vi "Panel DPT Channel Test Labels.vi"(5 "CDAQ?":bool) -> (6 "Chanel List":string="1001,1002,1003", 8 "Label Array":string[](array[string])=["RDB F", "Room Ambient(F)", "Tscale"], 10 "Pannel Array":string[](array[string])=["1-1", "1-2", "1-3"])   [LabVIEW 2012]
uses:
  DPT Channel Label.ctl
  <vilib>/Utility/file.llb/Write To Spreadsheet File (string).vi
  <vilib>/Utility/file.llb/Read From Spreadsheet File (string).vi
panel:
  out "error out":errorcluster={"status"=TRUE, "code"=1, "source"="Set Permissions in Panel DPT Channel Test Labels.vi<APPEND>\n<Not A Path>"}
  in  "TC Panel 4":T1[][](array[typedef])=[[{"Label"="", "Chan"="2021", "Rec"=FALSE, "TC Label"="1"}, {"Label"="", "Chan"="2022", "Rec"=FALSE, "TC Label"="2"}, {"Label"="", "Chan"="2023", "Rec"=FALSE, "TC Label"="3"}, {"Label"="", "Chan"="2024", "Rec"=FALSE, "TC Label"="4"}, {"Label"="", "Chan"="2025", "Rec"=FALSE, "TC Label"="5"}, {"Label"="", "Chan"="2026", "Rec"=FALSE, "TC Label"="6"}], [{"Label"="", "Chan"="2027", "Rec"=FALSE, "TC Label"="7"}, {"Label"="", "Chan"="2028", "Rec"=FALSE, "TC Label"="8"}, {"Label"="", "Chan"="2029", "Rec"=FALSE, "TC Label"="9"}, {"Label"="", "Chan"="2030", "Rec"=FALSE, "TC Label"="10"}, {"Label"="", "Chan"="2031", "Rec"=FALSE, "TC Label"="11"}, {"Label"="", "Chan"="2032", "Rec"=FALSE, "TC Label"="12"}], [{"Label"="", "Chan"="2033", "Rec"=FALSE, "TC Label"="13"}, {"Label"="", "Chan"="2034", "Rec"=FALSE, "TC Label"="14"}, {"Label"="", "Chan"="2035", "Rec"=FALSE, "TC Label"="15"}, {"Label"="", "Chan"="2036", "Rec"=FALSE, "TC Label"="16"}, {"Label"="", "Chan"="2037", "Rec"=FALSE, "TC Label"="17"}, {"Label"="", "Chan"="2038", "Rec"=FALSE, "TC Label"="18"}]]
  in  "Read":bool
  in  "Write":bool
  in  "Sensor 4":T1={"Label"="", "Chan"="", "Rec"=FALSE, "TC Label"="1"}
  in  "Read None":bool
  in  "Initialize":bool
  in  "Complete":bool
  in  "TC Panel 3":T1[][](array[typedef])=[[{"Label"="", "Chan"="2001", "Rec"=FALSE, "TC Label"="1"}, {"Label"="", "Chan"="2002", "Rec"=FALSE, "TC Label"="2"}, {"Label"="", "Chan"="2003", "Rec"=FALSE, "TC Label"="3"}, {"Label"="", "Chan"="2004", "Rec"=FALSE, "TC Label"="4"}, {"Label"="", "Chan"="2005", "Rec"=FALSE, "TC Label"="5"}, {"Label"="", "Chan"="2006", "Rec"=FALSE, "TC Label"="6"}], [{"Label"="", "Chan"="2007", "Rec"=FALSE, "TC Label"="7"}, {"Label"="", "Chan"="2008", "Rec"=FALSE, "TC Label"="8"}, {"Label"="", "Chan"="2009", "Rec"=FALSE, "TC Label"="9"}, {"Label"="", "Chan"="2010", "Rec"=FALSE, "TC Label"="10"}, {"Label"="", "Chan"="2011", "Rec"=FALSE, "TC Label"="11"}, {"Label"="", "Chan"="2012", "Rec"=FALSE, "TC Label"="12"}], [{"Label"="", "Chan"="2013", "Rec"=FALSE, "TC Label"="13"}, {"Label"="", "Chan"="2014", "Rec"=FALSE, "TC Label"="14"}, {"Label"="", "Chan"="2015", "Rec"=FALSE, "TC Label"="15"}, {"Label"="", "Chan"="2016", "Rec"=FALSE, "TC Label"="16"}, {"Label"="", "Chan"="2017", "Rec"=FALSE, "TC Label"="17"}, {"Label"="", "Chan"="2018", "Rec"=FALSE, "TC Label"="18"}]]
  in  "TC Panel 2":T1[][](array[typedef])=[[{"Label"="", "Chan"="1021", "Rec"=FALSE, "TC Label"="1"}, {"Label"="", "Chan"="1022", "Rec"=FALSE, "TC Label"="2"}, {"Label"="", "Chan"="1023", "Rec"=FALSE, "TC Label"="3"}, {"Label"="", "Chan"="1024", "Rec"=FALSE, "TC Label"="4"}, {"Label"="", "Chan"="1025", "Rec"=FALSE, "TC Label"="5"}, {"Label"="", "Chan"="1026", "Rec"=FALSE, "TC Label"="6"}], [{"Label"="", "Chan"="1027", "Rec"=FALSE, "TC Label"="7"}, {"Label"="", "Chan"="1028", "Rec"=FALSE, "TC Label"="8"}, {"Label"="", "Chan"="1029", "Rec"=FALSE, "TC Label"="9"}, {"Label"="", "Chan"="1030", "Rec"=FALSE, "TC Label"="10"}, {"Label"="", "Chan"="1031", "Rec"=FALSE, "TC Label"="11"}, {"Label"="", "Chan"="1032", "Rec"=FALSE, "TC Label"="12"}], [{"Label"="", "Chan"="1033", "Rec"=FALSE, "TC Label"="13"}, {"Label"="", "Chan"="1034", "Rec"=FALSE, "TC Label"="14"}, {"Label"="", "Chan"="1035", "Rec"=FALSE, "TC Label"="15"}, {"Label"="", "Chan"="1036", "Rec"=FALSE, "TC Label"="16"}, {"Label"="", "Chan"="1037", "Rec"=FALSE, "TC Label"="17"}, {"Label"="", "Chan"="1038", "Rec"=FALSE, "TC Label"="18"}]]
  in  "TC Panel 1":T1[][](array[typedef])=[[{"Label"="RDB F", "Chan"="1001", "Rec"=TRUE, "TC Label"="1"}, {"Label"="Room Ambient(F)", "Chan"="1002", "Rec"=TRUE, "TC Label"="2"}, {"Label"="Tscale", "Chan"="1003", "Rec"=TRUE, "TC Label"="3"}, {"Label"="", "Chan"="1004", "Rec"=FALSE, "TC Label"="4"}, {"Label"="", "Chan"="1005", "Rec"=FALSE, "TC Label"="5"}, {"Label"="", "Chan"="1006", "Rec"=FALSE, "TC Label"="6"}], [{"Label"="", "Chan"="1007", "Rec"=FALSE, "TC Label"="7"}, {"Label"="", "Chan"="1008", "Rec"=FALSE, "TC Label"="8"}, {"Label"="", "Chan"="1009", "Rec"=FALSE, "TC Label"="9"}, {"Label"="", "Chan"="1010", "Rec"=FALSE, "TC Label"="10"}, {"Label"="", "Chan"="1011", "Rec"=FALSE, "TC Label"="11"}, {"Label"="", "Chan"="1012", "Rec"=FALSE, "TC Label"="12"}], [{"Label"="", "Chan"="1013", "Rec"=FALSE, "TC Label"="13"}, {"Label"="", "Chan"="1014", "Rec"=FALSE, "TC Label"="14"}, {"Label"="", "Chan"="1015", "Rec"=FALSE, "TC Label"="15"}, {"Label"="", "Chan"="1016", "Rec"=FALSE, "TC Label"="16"}, {"Label"="", "Chan"="1017", "Rec"=FALSE, "TC Label"="17"}, {"Label"="", "Chan"="1018", "Rec"=FALSE, "TC Label"="18"}]]
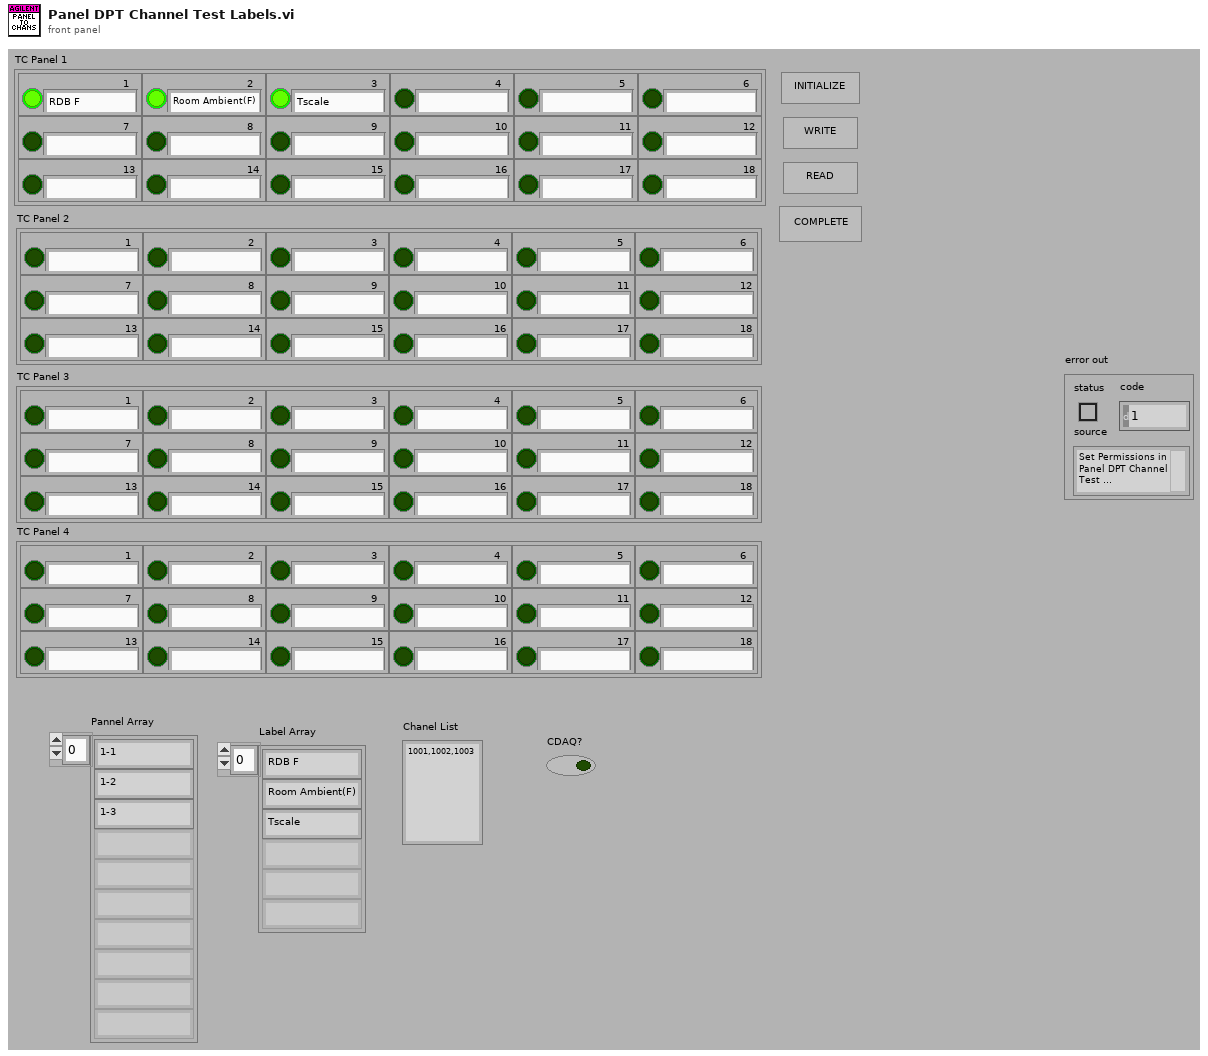
[diagram p1: front panel]
types:
  T1 = typedef "DPT Channel Label.ctl" = cluster{"Label":string, "Chan":string, "Rec":bool, "TC Label":string}
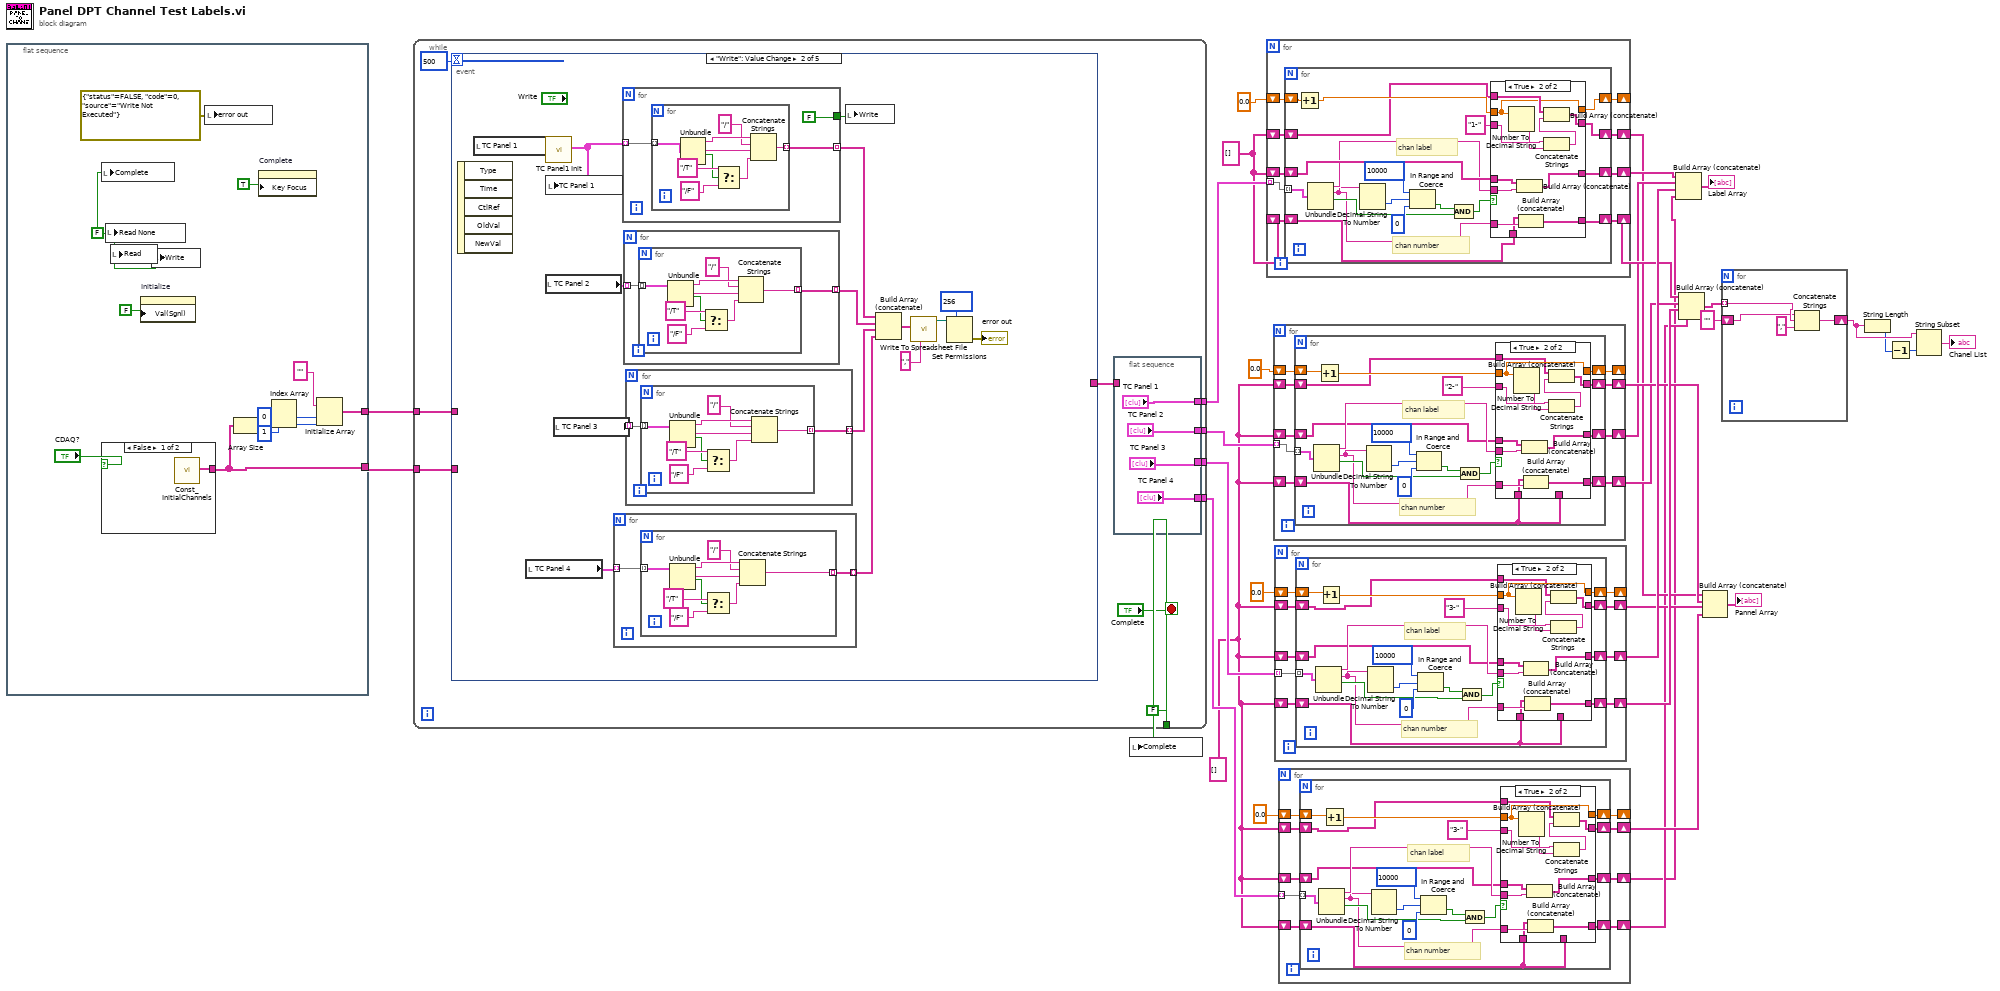
[diagram p0: block diagram]
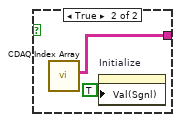
[diagram p4: hidden frame]
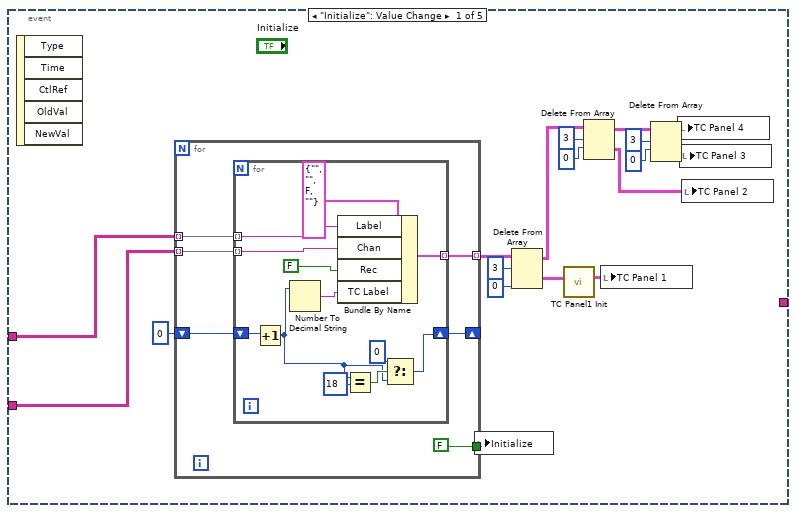
[diagram p7: hidden frame]
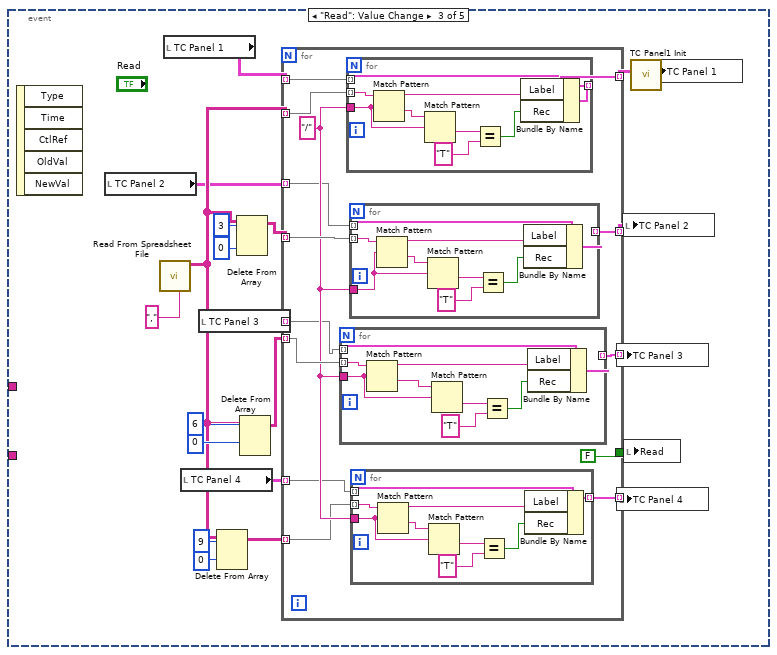
[diagram p8: hidden frame]
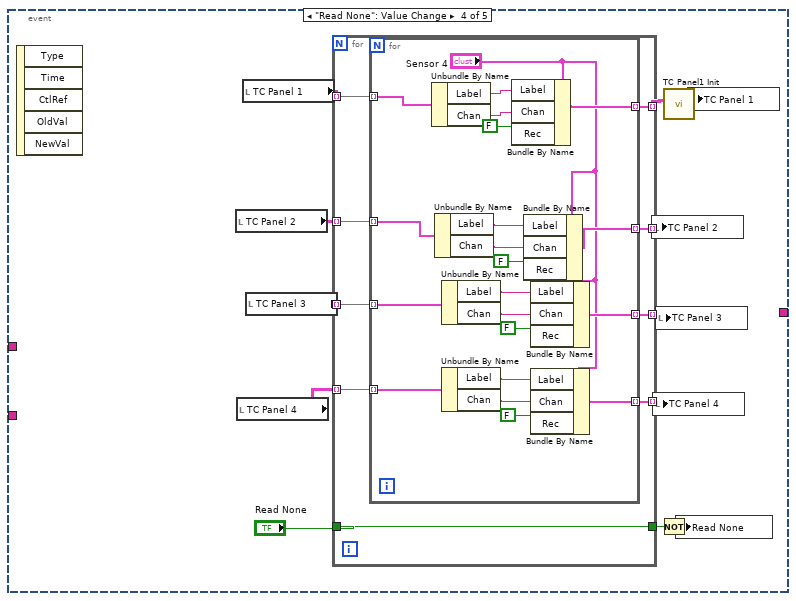
[diagram p9: hidden frame]
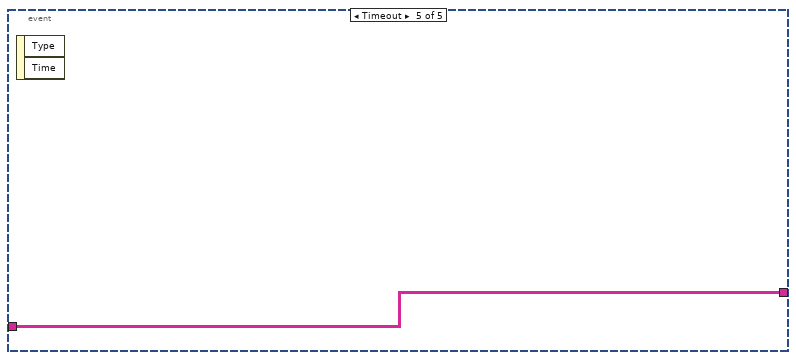
[diagram p10: hidden frame]
diagram:
  w3 = string[] []
  w9 = string[] []
  n1 = flat-sequence {
    tunnel: [w45] -> w33
    tunnel: [w38] -> w7
    frame #0 {
      w46 = FALSE ("Read None")
      n2 = local write "Complete"(w46) -> ()
      n3 = case shown="False" "CDAQ?" {
        tunnel: [w47 w49] -> w45
        frame False {
          n4 = call "Const_InitialChannels.vi"() -> ("appended array"=w47:string[][])  [unwired: 11 in]
        }
        frame True {
          n5 = call "CDAQ Index Array.vi"() -> ("CDAQ Index"=w49:string[][])  [unwired: 10 in]
          n6 = property on="Initialize" class="Bool (strict)"("Val(Sgnl)"=TRUE ("Value (Signaling)")) -> ()  [unwired: 2 in, 2 out]
        }
      }
      n7 = local write "Read None"(w46) -> ()
      n8 = local write "Read"(w46) -> ()
      n9 = property on="Initialize" class="Bool (strict)"("Val(Sgnl)"=FALSE ("Value (Signaling)")) -> ()  [unwired: 2 in, 2 out]
      n10 = local write "Write"(w46) -> ()
      n11 = local write "error out"(errorcluster {"status"=FALSE, "code"=0, "source"="Write Not Executed"} ("error out")) -> ()
      n12 = Array Size(array=w45) -> (size(s)=w44:i32[])
      n13 = property on="Complete" class="Bool (strict)"("Key Focus"=TRUE) -> ()  [unwired: 2 in, 2 out]
      n14 = Index Array(array=w44, index #1=0 ("index"), index #2=1 ("index")) -> (element #1=w41:i32, element #2=w40:i32)
      n15 = Initialize Array("", w41, w40) -> (w38:string[][])
    }
  }
  n16 = while {
    tunnel: w7 -> [w59]
    tunnel: w33 -> [w58]
    tunnel: [w56] -> w32
    tunnel: [w55] -> w12
    tunnel: [w54] -> w31
    tunnel: [FALSE ("Read None")] -> w25
    tunnel: [w51] -> w4
    stop <- "Complete" stop-if-true
    n17 = event shown="[1] \"Write\": Value Change" {
      selector: _ -> [_ _ _ _ _]
      dyn-events: _ -> [_ _ _ _ _]
      timeout: 500 -> [_ _ _ _ _]
      tunnel: w59 -> [w81 _ _ _ w273]
      tunnel: w58 -> [w80 _ _ _ _]
      tunnel: [_ _ _ _ w273] -> w50
      event "Initialize": Value Change {
        n18 = event-data() -> ()  [unwired: 1 in, 5 out]
        n19 = for {
          tunnel: [w87] -> w79 mode=indexing
          tunnel: w81 -> [w86] mode=indexing
          tunnel: w80 -> [w85] mode=indexing
          tunnel: [FALSE ("Read None")] -> w72
          shift-right: [w82] -> _
          shift-left: 0 -> [w83]
          n20 = for {
            tunnel: [w99] -> w87 mode=indexing
            tunnel: w86 -> [w98] mode=indexing
            tunnel: w85 -> [w97] mode=indexing
            shift-right: [w88] -> w82
            shift-left: w83 -> [w93]
            n21 = Increment(x=w93) -> (x+1=w90:i32)
            n22 = Number To Decimal String(number=w90) -> (decimal integer string=w94:string)  [unwired: 1 in]
            n23 = Bundle By Name(cluster=T1 {"Label"="", "Chan"="", "Rec"=FALSE, "TC Label"=""} ("Sensor 2"), "Label"=w98, "Chan"=w97, "Rec"=FALSE, "TC Label"=w94) -> (w99:T1)
            n24 = Equal?(x=w90, y=18) -> (x = y?=w91:bool)
            n25 = Select(t=0, s=w91, f=w90) -> (s? t:f=w88:i32)
          }
        }
        n26 = local write "Initialize"(w72) -> ()
        n27 = Delete From Array(array=w79, length=3, index (row)=0) -> (deleted portion=w65:T1[][], array with subset deleted=w74:T1[][])  [unwired: 1 in]
        n28 = call "TC Panel1 Init.vi"("TC Panel 1"=w65) -> ("TC Panel 1 Out"=w66:T1[][])  [unwired: 10 in]
        n29 = Delete From Array(array=w74, length=3, index (row)=0) -> (deleted portion=w73:T1[][], array with subset deleted=w69:T1[][])  [unwired: 1 in]
        n30 = local write "TC Panel 1"(w66) -> ()
        n31 = Delete From Array(array=w69, length=3, index (row)=0) -> (deleted portion=w68:T1[][], array with subset deleted=w67:T1[][])  [unwired: 1 in]
        n32 = local write "TC Panel 4"(w67) -> ()
        n33 = local write "TC Panel 3"(w68) -> ()
        n34 = local write "TC Panel 2"(w73) -> ()
      }
      event "Write": Value Change {
        n35 = event-data() -> ()  [unwired: 1 in, 5 out]
        n36 = local read "TC Panel 1"() -> (w113:T1[][])
        n37 = local read "TC Panel 4"() -> (w106:T1[][])
        n38 = local read "TC Panel 2"() -> (w111:T1[][])
        n39 = call "TC Panel1 Init.vi"("TC Panel 1"=w113) -> ("TC Panel 1 Out"=w104:T1[][])  [unwired: 10 in]
        n40 = local write "TC Panel 1"(w104) -> ()
        n41 = local read "TC Panel 3"() -> (w110:T1[][])
        n42 = for {
          tunnel: w106 -> [w116] mode=indexing
          tunnel: [w115] -> w105 mode=indexing
          n43 = for {
            tunnel: w116 -> [w125] mode=indexing
            tunnel: [w117] -> w115 mode=indexing
            n44 = Unbundle(w125) -> ("Label"=w124:string, "Chan"=w122:string, "Rec"=w119:bool)  [unwired: 1 out]
            n45 = Select(t="/T" ("string"), s=w119, f="/F" ("string")) -> (s? t:f=w118:string)
            n46 = Concatenate Strings(w124, "/" ("string"), w122, w118) -> (w117:string)
          }
        }
        n47 = for {
          tunnel: w104 -> [w150] mode=indexing
          tunnel: [FALSE ("Read None")] -> w114
          tunnel: [w148] -> w109 mode=indexing
          n48 = for {
            tunnel: w150 -> [w159] mode=indexing
            tunnel: [w151] -> w148 mode=indexing
            n49 = Unbundle(w159) -> ("Label"=w158:string, "Chan"=w156:string, "Rec"=w153:bool)  [unwired: 1 out]
            n50 = Select(t="/T" ("string"), s=w153, f="/F" ("string")) -> (s? t:f=w152:string)
            n51 = Concatenate Strings(w158, "/" ("string"), w156, w152) -> (w151:string)
          }
        }
        n52 = for {
          tunnel: w111 -> [w138] mode=indexing
          tunnel: [w137] -> w108 mode=indexing
          n53 = for {
            tunnel: w138 -> [w147] mode=indexing
            tunnel: [w139] -> w137 mode=indexing
            n54 = Unbundle(w147) -> ("Label"=w146:string, "Chan"=w144:string, "Rec"=w141:bool)  [unwired: 1 out]
            n55 = Select(t="/T" ("string"), s=w141, f="/F" ("string")) -> (s? t:f=w140:string)
            n56 = Concatenate Strings(w146, "/" ("string"), w144, w140) -> (w139:string)
          }
        }
        n57 = for {
          tunnel: w110 -> [w127] mode=indexing
          tunnel: [w126] -> w107 mode=indexing
          n58 = for {
            tunnel: w127 -> [w136] mode=indexing
            tunnel: [w128] -> w126 mode=indexing
            n59 = Unbundle(w136) -> ("Label"=w135:string, "Chan"=w133:string, "Rec"=w130:bool)  [unwired: 1 out]
            n60 = Select(t="/T" ("string"), s=w130, f="/F" ("string")) -> (s? t:f=w129:string)
            n61 = Concatenate Strings(w135, "/" ("string"), w133, w129) -> (w128:string)
          }
        }
        n62 = local write "Write"(w114) -> ()
        n63 = Build Array (concatenate)(w109, w108, w107, w105) -> (w100:string[][])
        n64 = call-poly <vilib>:"Write To Spreadsheet File.vi"("delimiter (\\t)"="," ("delimiter (\\t)"), "2D data"=w100) -> ("new file path (Not A Path if cancelled)"=w103:path)  [unwired: 6 in]
        n65 = Set Permissions(7:i16 256 ("permissions"), 11:w103) -> (0:→"error out":errorcluster)  [unwired: 3 in, 1 out]
      }
      event "Read": Value Change {
        n66 = event-data() -> ()  [unwired: 1 in, 5 out]
        n67 = local read "TC Panel 2"() -> (w162:T1[][])
        n68 = call-poly <vilib>:"Read From Spreadsheet File.vi"("delimiter (\\t)"="," ("delimiter (\\t)")) -> ("all rows"=w166:string[][])  [unwired: 6 in, 4 out]
        n69 = local read "TC Panel 1"() -> (w171:T1[][])
        n70 = local read "TC Panel 4"() -> (w160:T1[][])
        n71 = local read "TC Panel 3"() -> (w161:T1[][])
        n72 = Delete From Array(array=w166, length=9, index (row)=0) -> (array with subset deleted=w165:string[][])  [unwired: 1 in, 1 out]
        n73 = Delete From Array(array=w166, length=3, index (row)=0) -> (array with subset deleted=w175:string[][])  [unwired: 1 in, 1 out]
        n74 = Delete From Array(array=w166, length=6, index (row)=0) -> (array with subset deleted=w176:string[][])  [unwired: 1 in, 1 out]
        n75 = for {
          tunnel: w171 -> [w185] mode=indexing
          tunnel: w166 -> [w194] mode=indexing
          tunnel: [w193] -> w174 mode=indexing
          tunnel: w175 -> [w192] mode=indexing
          tunnel: w176 -> [w189] mode=indexing
          tunnel: [w191] -> w173 mode=indexing
          tunnel: [w190] -> w172 mode=indexing
          tunnel: [FALSE ("Read")] -> w170
          tunnel: w165 -> [w186] mode=indexing
          tunnel: [w184] -> w164 mode=indexing
          tunnel: w162 -> [w183] mode=indexing
          tunnel: w161 -> [w182] mode=indexing
          tunnel: w160 -> [w181] mode=indexing
          w187 = "/" ("regular expression")
          n76 = for {
            tunnel: w182 -> [w211] mode=indexing
            tunnel: w189 -> [w212] mode=indexing
            tunnel: [w209] -> w190 mode=indexing
            tunnel: w187 -> [w204]
            n77 = Match Pattern(string=w212, regular expression=w204) -> (before substring=w210:string, after substring=w208:string)  [unwired: 1 in, 2 out]
            n78 = Match Pattern(string=w208, regular expression=w204) -> (after substring=w207:string)  [unwired: 1 in, 3 out]
            n79 = Equal?(x=w207, y="T") -> (x = y?=w205:bool)
            n80 = Bundle By Name(cluster=w211, "Label"=w210, "Rec"=w205) -> (w209:T1)
          }
          n81 = for {
            tunnel: w185 -> [w229] mode=indexing
            tunnel: w194 -> [w230] mode=indexing
            tunnel: [w227] -> w193 mode=indexing
            tunnel: w187 -> [w222]
            n82 = Match Pattern(string=w230, regular expression=w222) -> (before substring=w228:string, after substring=w226:string)  [unwired: 1 in, 2 out]
            n83 = Match Pattern(string=w226, regular expression=w222) -> (after substring=w225:string)  [unwired: 1 in, 3 out]
            n84 = Equal?(x=w225, y="T") -> (x = y?=w223:bool)
            n85 = Bundle By Name(cluster=w229, "Label"=w228, "Rec"=w223) -> (w227:T1)
          }
          n86 = for {
            tunnel: w183 -> [w220] mode=indexing
            tunnel: w192 -> [w221] mode=indexing
            tunnel: [w218] -> w191 mode=indexing
            tunnel: w187 -> [w213]
            n87 = Match Pattern(string=w221, regular expression=w213) -> (before substring=w219:string, after substring=w217:string)  [unwired: 1 in, 2 out]
            n88 = Match Pattern(string=w217, regular expression=w213) -> (after substring=w216:string)  [unwired: 1 in, 3 out]
            n89 = Equal?(x=w216, y="T") -> (x = y?=w214:bool)
            n90 = Bundle By Name(cluster=w220, "Label"=w219, "Rec"=w214) -> (w218:T1)
          }
          n91 = for {
            tunnel: w181 -> [w202] mode=indexing
            tunnel: w186 -> [w203] mode=indexing
            tunnel: [w200] -> w184 mode=indexing
            tunnel: w187 -> [w195]
            n92 = Match Pattern(string=w203, regular expression=w195) -> (before substring=w201:string, after substring=w199:string)  [unwired: 1 in, 2 out]
            n93 = Match Pattern(string=w199, regular expression=w195) -> (after substring=w198:string)  [unwired: 1 in, 3 out]
            n94 = Equal?(x=w198, y="T") -> (x = y?=w196:bool)
            n95 = Bundle By Name(cluster=w202, "Label"=w201, "Rec"=w196) -> (w200:T1)
          }
        }
        n96 = local write "TC Panel 3"(w172) -> ()
        n97 = local write "TC Panel 4"(w164) -> ()
        n98 = local write "TC Panel 2"(w173) -> ()
        n99 = local write "Read"(w170) -> ()
        n100 = call "TC Panel1 Init.vi"("TC Panel 1"=w174) -> ("TC Panel 1 Out"=w163:T1[][])  [unwired: 10 in]
        n101 = local write "TC Panel 1"(w163) -> ()
      }
      event "Read None": Value Change {
        n102 = event-data() -> ()  [unwired: 1 in, 5 out]
        n103 = local read "TC Panel 2"() -> (w239:T1[][])
        n104 = local read "TC Panel 4"() -> (w233:T1[][])
        n105 = local read "TC Panel 1"() -> (w242:T1[][])
        n106 = local read "TC Panel 3"() -> (w238:T1[][])
        n107 = for {
          tunnel: [w251] -> w241 mode=indexing
          tunnel: w242 -> [w250] mode=indexing
          tunnel: [w249] -> w240 mode=indexing
          tunnel: w239 -> [w248] mode=indexing
          tunnel: w238 -> [w247] mode=indexing
          tunnel: [w246] -> w237 mode=indexing
          tunnel: [w245] -> w235
          tunnel: "Read None" -> [w245]
          tunnel: w233 -> [w244] mode=indexing
          tunnel: [w243] -> w232 mode=indexing
          n108 = for {
            tunnel: [w272] -> w251 mode=indexing
            tunnel: w250 -> [w271] mode=indexing
            tunnel: [w267] -> w249 mode=indexing
            tunnel: w248 -> [w266] mode=indexing
            tunnel: w247 -> [w262] mode=indexing
            tunnel: [w261] -> w246 mode=indexing
            tunnel: w244 -> [w256] mode=indexing
            tunnel: [w255] -> w243 mode=indexing
            n109 = Unbundle By Name(w271) -> ("Label"=w253:string, "Chan"=w252:string)
            n110 = Unbundle By Name(w266) -> ("Label"=w269:string, "Chan"=w270:string)
            n111 = Unbundle By Name(w262) -> ("Label"=w264:string, "Chan"=w263:string)
            n112 = Unbundle By Name(w256) -> ("Label"=w259:string, "Chan"=w260:string)
            n113 = Bundle By Name(cluster="Sensor 4", "Label"=w253, "Chan"=w252, "Rec"=FALSE) -> (w272:T1)
            n114 = Bundle By Name(cluster="Sensor 4", "Label"=w269, "Chan"=w270, "Rec"=FALSE) -> (w267:T1)
            n115 = Bundle By Name(cluster="Sensor 4", "Label"=w264, "Chan"=w263, "Rec"=FALSE) -> (w261:T1)
            n116 = Bundle By Name(cluster="Sensor 4", "Label"=w259, "Chan"=w260, "Rec"=FALSE) -> (w255:T1)
          }
        }
        n117 = local write "TC Panel 2"(w240) -> ()
        n118 = local write "TC Panel 4"(w232) -> ()
        n119 = local write "TC Panel 3"(w237) -> ()
        n120 = Not(x=w235) -> (.not. x?=w236:bool)
        n121 = call "TC Panel1 Init.vi"("TC Panel 1"=w241) -> ("TC Panel 1 Out"=w231:T1[][])  [unwired: 10 in]
        n122 = local write "Read None"(w236) -> ()
        n123 = local write "TC Panel 1"(w231) -> ()
      }
      event Timeout {
        n124 = event-data() -> ()  [unwired: 1 in, 2 out]
      }
    }
    n125 = flat-sequence {
      tunnel: ["TC Panel 1"] -> w56
      tunnel: ["TC Panel 2"] -> w55
      tunnel: ["TC Panel 3"] -> w54
      tunnel: ["TC Panel 4"] -> w51
      tunnel: w50 -> [_]
      frame #0 {
      }
    }
  }
  n126 = local write "Complete"(w25) -> ()
  n127 = for {
    tunnel: w32 -> [w282] mode=indexing
    shift-right: [w281] -> w30
    shift-left: w9 -> [w280]
    shift-right: [w279] -> w26
    shift-left: w9 -> [w278]
    shift-right: [w276] -> _
    shift-left: 0.0 -> [w277]
    shift-right: [w274] -> w8
    shift-left: w9 -> [w275]
    n128 = for {
      tunnel: w282 -> [w301] mode=indexing
      shift-right: [w294] -> w281
      shift-left: w280 -> [w288]
      shift-right: [w284] -> w279
      shift-left: w278 -> [w285]
      shift-right: [w293] -> w276
      shift-left: w277 -> [w295]
      shift-right: [w290] -> w274
      shift-left: w275 -> [w291]
      # "chan label"
      # "chan number"
      n129 = Increment(x=w295) -> (x+1=w292:dbl)
      n130 = Unbundle(w301) -> ("Label"=w287:string, "Chan"=w286:string, "Rec"=w296:bool)  [unwired: 1 out]
      n131 = Decimal String To Number(string=w286) -> (number=w300:i32)  [unwired: 2 in, 1 out]
      n132 = In Range and Coerce(upper limit=10000, x=w300, lower limit=0) -> (In Range?=w297:bool)  [unwired: 1 out]
      n133 = Compound Arithmetic op=AND(w297, w296) -> (w289:bool)
      n134 = case shown="True" w289 {
        tunnel: w287 -> [_ w317]
        tunnel: [w305 w316] -> w294
        tunnel: w288 -> [w305 w314]
        tunnel: [w302 w315] -> w284
        tunnel: w286 -> [_ w313]
        tunnel: w285 -> [w302 w312]
        tunnel: w292 -> [w304 w306]
        tunnel: [w303 w311] -> w290
        tunnel: [w304 w306] -> w293
        tunnel: "1-" -> [_ w310]
        tunnel: w291 -> [w303 w307]
        frame False {
        }
        frame True {
          n135 = Number To Decimal String(number=w306) -> (decimal integer string=w309:string)  [unwired: 1 in]
          n136 = Build Array (concatenate)(w314, w317) -> (w316:string[])
          n137 = Build Array (concatenate)(w312, w313) -> (w315:string[])
          n138 = Concatenate Strings(w310, w309) -> (w308:string)
          n139 = Build Array (concatenate)(w307, w308) -> (w311:string[])
        }
      }
    }
  }
  n140 = for {
    tunnel: w12 -> [w326] mode=indexing
    shift-right: [w325] -> w10
    shift-left: w3 -> [w324]
    shift-right: [w323] -> w11
    shift-left: w3 -> [w322]
    shift-right: [w319] -> _
    shift-left: 0.0 -> [w321]
    shift-right: [w320] -> w13
    shift-left: w3 -> [w318]
    n141 = for {
      tunnel: w326 -> [w345] mode=indexing
      shift-right: [w338] -> w325
      shift-left: w324 -> [w337]
      shift-right: [w335] -> w323
      shift-left: w322 -> [w333]
      shift-right: [w329] -> w319
      shift-left: w321 -> [w332]
      shift-right: [w330] -> w320
      shift-left: w318 -> [w327]
      # "chan label"
      # "chan number"
      n142 = Unbundle(w345) -> ("Label"=w339:string, "Chan"=w334:string, "Rec"=w340:bool)  [unwired: 1 out]
      n143 = Increment(x=w332) -> (x+1=w331:dbl)
      n144 = Decimal String To Number(string=w334) -> (number=w344:i32)  [unwired: 2 in, 1 out]
      n145 = In Range and Coerce(upper limit=10000, x=w344, lower limit=0) -> (In Range?=w341:bool)  [unwired: 1 out]
      n146 = And(x=w341, y=w340) -> (x .and. y?=w336:bool)
      n147 = case shown="True" w336 {
        tunnel: w339 -> [_ w361]
        tunnel: [w349 w360] -> w338
        tunnel: w337 -> [w349 w358]
        tunnel: [w348 w359] -> w335
        tunnel: w334 -> [_ w357]
        tunnel: w333 -> [w348 _]
        tunnel: w333 -> [_ w356]
        tunnel: w331 -> [w347 w354]
        tunnel: [w346 w355] -> w330
        tunnel: [w347 w354] -> w329
        tunnel: "2-" -> [_ w353]
        tunnel: w327 -> [w346 w350]
        frame False {
        }
        frame True {
          n148 = Number To Decimal String(number=w354) -> (decimal integer string=w352:string)  [unwired: 1 in]
          n149 = Build Array (concatenate)(w358, w361) -> (w360:string[])
          n150 = Build Array (concatenate)(w356, w357) -> (w359:string[])
          n151 = Concatenate Strings(w353, w352) -> (w351:string)
          n152 = Build Array (concatenate)(w350, w351) -> (w355:string[])
        }
      }
    }
  }
  n153 = for {
    tunnel: w31 -> [w370] mode=indexing
    shift-right: [w369] -> w29
    shift-left: w3 -> [w368]
    shift-right: [w367] -> w27
    shift-left: w3 -> [w366]
    shift-right: [w363] -> _
    shift-left: 0.0 -> [w365]
    shift-right: [w364] -> w15
    shift-left: w3 -> [w362]
    n154 = for {
      tunnel: w370 -> [w389] mode=indexing
      shift-right: [w382] -> w369
      shift-left: w368 -> [w381]
      shift-right: [w379] -> w367
      shift-left: w366 -> [w377]
      shift-right: [w373] -> w363
      shift-left: w365 -> [w376]
      shift-right: [w374] -> w364
      shift-left: w362 -> [w371]
      # "chan label"
      # "chan number"
      n155 = Unbundle(w389) -> ("Label"=w383:string, "Chan"=w378:string, "Rec"=w384:bool)  [unwired: 1 out]
      n156 = Increment(x=w376) -> (x+1=w375:dbl)
      n157 = Decimal String To Number(string=w378) -> (number=w388:i32)  [unwired: 2 in, 1 out]
      n158 = In Range and Coerce(upper limit=10000, x=w388, lower limit=0) -> (In Range?=w385:bool)  [unwired: 1 out]
      n159 = And(x=w385, y=w384) -> (x .and. y?=w380:bool)
      n160 = case shown="True" w380 {
        tunnel: w383 -> [_ w405]
        tunnel: [w393 w404] -> w382
        tunnel: w381 -> [w393 w402]
        tunnel: [w392 w403] -> w379
        tunnel: w378 -> [_ w401]
        tunnel: w377 -> [w392 _]
        tunnel: w377 -> [_ w400]
        tunnel: w375 -> [w391 w398]
        tunnel: [w390 w399] -> w374
        tunnel: [w391 w398] -> w373
        tunnel: "3-" -> [_ w397]
        tunnel: w371 -> [w390 w394]
        frame False {
        }
        frame True {
          n161 = Number To Decimal String(number=w398) -> (decimal integer string=w396:string)  [unwired: 1 in]
          n162 = Build Array (concatenate)(w402, w405) -> (w404:string[])
          n163 = Build Array (concatenate)(w400, w401) -> (w403:string[])
          n164 = Concatenate Strings(w397, w396) -> (w395:string)
          n165 = Build Array (concatenate)(w394, w395) -> (w399:string[])
        }
      }
    }
  }
  n166 = for {
    tunnel: w4 -> [w414] mode=indexing
    shift-right: [w413] -> w1
    shift-left: w3 -> [w412]
    shift-right: [w411] -> w2
    shift-left: w3 -> [w410]
    shift-right: [w407] -> _
    shift-left: 0.0 -> [w409]
    shift-right: [w408] -> w5
    shift-left: w3 -> [w406]
    n167 = for {
      tunnel: w414 -> [w433] mode=indexing
      shift-right: [w426] -> w413
      shift-left: w412 -> [w425]
      shift-right: [w423] -> w411
      shift-left: w410 -> [w421]
      shift-right: [w417] -> w407
      shift-left: w409 -> [w420]
      shift-right: [w418] -> w408
      shift-left: w406 -> [w415]
      # "chan label"
      # "chan number"
      n168 = Unbundle(w433) -> ("Label"=w427:string, "Chan"=w422:string, "Rec"=w428:bool)  [unwired: 1 out]
      n169 = Increment(x=w420) -> (x+1=w419:dbl)
      n170 = Decimal String To Number(string=w422) -> (number=w432:i32)  [unwired: 2 in, 1 out]
      n171 = In Range and Coerce(upper limit=10000, x=w432, lower limit=0) -> (In Range?=w429:bool)  [unwired: 1 out]
      n172 = And(x=w429, y=w428) -> (x .and. y?=w424:bool)
      n173 = case shown="True" w424 {
        tunnel: w427 -> [_ w449]
        tunnel: [w437 w448] -> w426
        tunnel: w425 -> [w437 w446]
        tunnel: [w436 w447] -> w423
        tunnel: w422 -> [_ w445]
        tunnel: w421 -> [w436 _]
        tunnel: w421 -> [_ w444]
        tunnel: w419 -> [w435 w442]
        tunnel: [w434 w443] -> w418
        tunnel: [w435 w442] -> w417
        tunnel: "3-" -> [_ w441]
        tunnel: w415 -> [w434 w438]
        frame False {
        }
        frame True {
          n174 = Number To Decimal String(number=w442) -> (decimal integer string=w440:string)  [unwired: 1 in]
          n175 = Build Array (concatenate)(w446, w449) -> (w448:string[])
          n176 = Build Array (concatenate)(w444, w445) -> (w447:string[])
          n177 = Concatenate Strings(w441, w440) -> (w439:string)
          n178 = Build Array (concatenate)(w438, w439) -> (w443:string[])
        }
      }
    }
  }
  n179 = Build Array (concatenate)(w30, w10, w29, w1) -> (→"Label Array":string[])
  n180 = Build Array (concatenate)(w26, w11, w27, w2) -> (w24:string[])
  n181 = Build Array (concatenate)(w8, w13, w15, w5) -> (→"Pannel Array":string[])
  n182 = for {
    tunnel: w24 -> [w452] mode=indexing
    shift-right: [w451] -> w22
    shift-left: "" -> [w450]
    n183 = Concatenate Strings(w450, w452, "," ("string")) -> (w451:string)
  }
  n184 = String Length(string=w22) -> (length=w20:i32)
  n185 = Decrement(x=w20) -> (x-1=w21:i32)
  n186 = String Subset(string=w22, length (rest)=w21) -> (substring=→"Chanel List":string)  [unwired: 1 in]
